vi "numCmd_Send_Internal.vi"(7 "Command Name":string, 11 "Value":variant) -> (0 "error out":errorcluster)   [LabVIEW 2019, in "Trajectory_Library.lvlib"]
uses:
  Trajectory_Library.lvlib
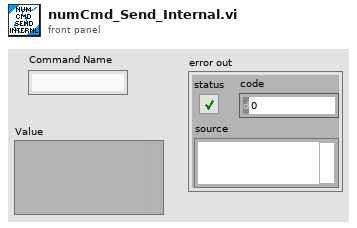
[diagram p1: front panel]
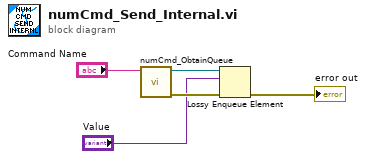
[diagram p0: block diagram]
diagram:
  n1 = call "numCmd_ObtainQueue.vi"("Command Name"="Command Name") -> ("error out"=w3:errorcluster, "queue out"=w4:refnum<queue>)  [unwired: 9 in]
  n2 = Lossy Enqueue Element(queue=w4, element="Value", error in (no error)=w3) -> (error out=→"error out":errorcluster)  [unwired: 3 out]
